vi "IX81 Parse Reply.vi"(7 "Reply In":string, 11 "Error In":errorcluster) -> (8 "Reply Out":string, 15 "Error Out":errorcluster)   [LabVIEW 2020]
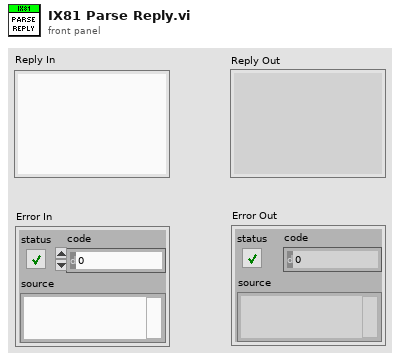
[diagram p1: front panel]
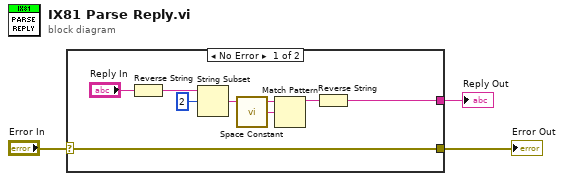
[diagram p0: block diagram]
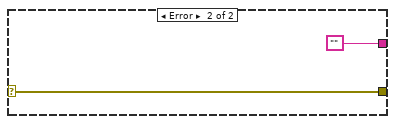
[diagram p2: hidden frame]
diagram:
  n1 = case shown="No Error" "Error In" {
    selector: "Error In" -> [w6 w13]
    tunnel: [w6 w13] -> w2
    tunnel: [w4 ""] -> w1
    frame No Error {
      n2 = Reverse String(1:"Reply In") -> (0:w11:string)
      n3 = String Subset(string=w11, offset (0)=2) -> (substring=w8:string)  [unwired: 1 in]
      n4 = call <vilib>:"Space Constant.vi"() -> ("String"=w7:string)
      n5 = Match Pattern(string=w8, regular expression=w7) -> (before substring=w5:string)  [unwired: 1 in, 3 out]
      n6 = Reverse String(1:w5) -> (0:w4:string)
    }
    frame Error {
    }
  }
  "Error Out" <- w2
  "Reply Out" <- w1
